vi "Batch file open.vi"(10 "file path (use dialog)":path) -> (2 "cmd":string[](array[string]))   [LabVIEW 2018]
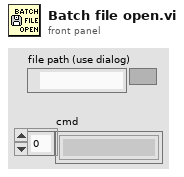
[diagram p1: front panel]
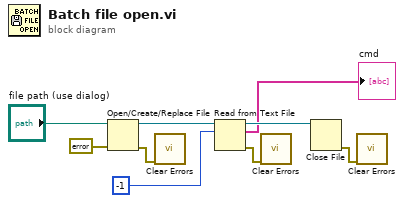
[diagram p0: block diagram]
diagram:
  n1 = Open/Create/Replace File(file path (use dialog)="file path (use dialog)", error in=errorcluster {"status"=FALSE, "code"=0, "source"=""}) -> (refnum out=w9:refnum<file>, error out=w3:errorcluster)  [unwired: 4 in, 1 out]
  n2 = call <vilib>:"Clear Errors.vi"("error in (no error)"=w3) -> ()  [unwired: 5 in, 2 out]
  n3 = Read from Text File(file (use dialog)=w9, count=-1) -> (refnum out=w8:refnum<file>, text=→"cmd":string[], error out=w2:errorcluster)  [unwired: 2 in, 1 out]
  n4 = call <vilib>:"Clear Errors.vi"("error in (no error)"=w2) -> ()  [unwired: 5 in, 2 out]
  n5 = Close File(refnum=w8) -> (error out=w1:errorcluster)  [unwired: 1 in, 1 out]
  n6 = call <vilib>:"Clear Errors.vi"("error in (no error)"=w1) -> ()  [unwired: 5 in, 2 out]
